vi "CPP_TubingCompGlobal.vi"() -> ()   [LabVIEW 2011]
panel:
  in  "Freq-BoostArray":dbl[][](array[numeric])
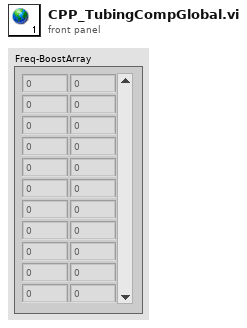
[diagram p1: front panel]
diagram:
